vi "LoadTachSettings.vi"(8 "error in (no error)":errorcluster, 11 "Tree DVR in":refnum<data-value>) -> (0 "error out":errorcluster, 3 "Tachometer Controls":T1)   [LabVIEW 2014]
uses:
  Controls/TachometerControls.ctl
  <vilib>/MDSplus/Classes/Tree_Class/Tree.lvclass
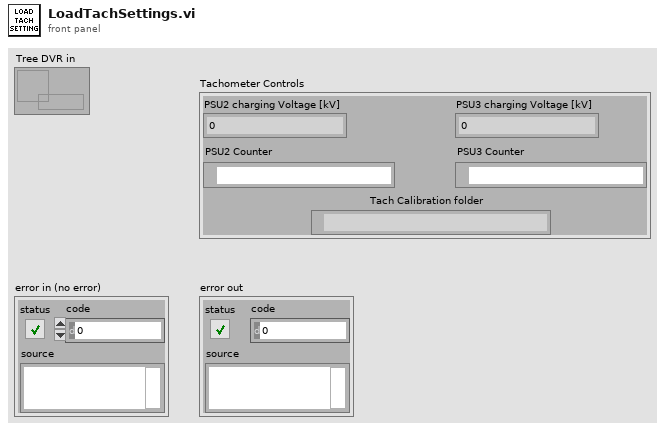
[diagram p1: front panel]
types:
  T1 = typedef "TachometerControls.ctl" = cluster{"Tach Calibration folder":path, "PSU2 charging Voltage [kV]":dbl, "PSU2 Counter":tag, "PSU3 Counter":tag, "PSU3 charging Voltage [kV]":dbl}
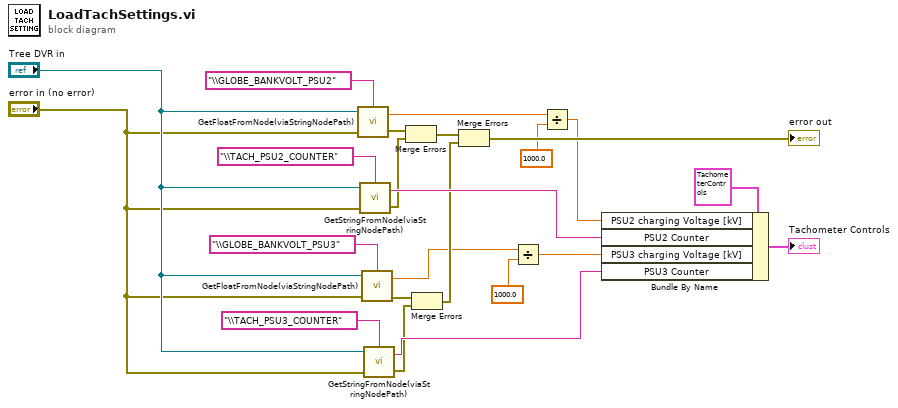
[diagram p0: block diagram]
diagram:
  n1 = call "GetFloatFromNode(viaStringNodePath).vi"("Path"="\\GLOBE_BANKVOLT_PSU2", "error in"="error in (no error)", "Tree DVR in"="Tree DVR in") -> ("error out"=w12:errorcluster, "Float64"=w6:dbl)  [unwired: 1 in]
  n2 = call "GetStringFromNode(viaStringNodePath).vi"("Path"="\\TACH_PSU2_COUNTER", "error in"="error in (no error)", "Tree DVR in"="Tree DVR in") -> ("error out"=w14:errorcluster, "String out"=w20:string)  [unwired: 1 in]
  n3 = call "GetFloatFromNode(viaStringNodePath).vi"("Path"="\\GLOBE_BANKVOLT_PSU3", "error in"="error in (no error)", "Tree DVR in"="Tree DVR in") -> ("error out"=w13:errorcluster, "Float64"=w2:dbl)  [unwired: 1 in]
  n4 = call "GetStringFromNode(viaStringNodePath).vi"("Path"="\\TACH_PSU3_COUNTER", "error in"="error in (no error)", "Tree DVR in"="Tree DVR in") -> ("error out"=w15:errorcluster, "String out"=w21:string)  [unwired: 1 in]
  n5 = Merge Errors(w12, w14) -> (w16:errorcluster)
  n6 = Merge Errors(w13, w15) -> (w17:errorcluster)
  n7 = Merge Errors(w16, w17) -> (→"error out":errorcluster)
  n8 = Divide(x=w2, y=1000.0) -> (x/y=w1:dbl)
  n9 = Divide(x=w6, y=1000.0) -> (x/y=w5:dbl)
  n10 = Bundle By Name(cluster=T1 {"Tach Calibration folder"=path "Z:/Data/Calibration/Tachometer", "PSU2 charging Voltage [kV]"=0.0, "PSU2 Counter"="", "PSU3 Counter"="", "PSU3 charging Voltage [kV]"=0.0} ("Tachometer Controls"), "PSU2 charging Voltage [kV]"=w5, "PSU2 Counter"=w20, "PSU3 charging Voltage [kV]"=w1, "PSU3 Counter"=w21) -> (→"Tachometer Controls":T1)
